vi "localEngineReference2.vi"   [LabVIEW 2017]
doc: "Use this constant to supply a reference to one of the following items:"
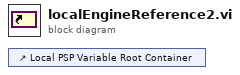
[diagram p0: block diagram]
diagram:
  n1 = control-ref of="Local PSP Variable Root Container"() -> ()  [unwired: 1 out]
